vi "setUp.vi"(8 "error in (no error)":errorcluster, 11 "reference in":refnum<class "Engine Simulation Multi FPGA System Tests.lvclass">) -> (0 "error out":errorcluster, 3 "reference out":refnum<class "Engine Simulation Multi FPGA System Tests.lvclass">)   [LabVIEW 2017, in "Engine Simulation Multi FPGA System Tests.lvclass"]
doc: "setUp runs prior to the test method during test execution. Use this method to initialize any object data required by your tests."
uses:
  Engine Simulation Multi FPGA System Tests.lvclass
  C:/Program Files (x86)/National Instruments/LabVIEW 2017/vi.lib/addons/_JKI Toolkits/VI Tester/TestCase.llb/TestCase.lvclass
  <vilib>/addons/_JKI Toolkits/VI Tester/TestCase.llb/TestCase.lvclass
panel:
  in  "Minimum VeriStand Version":string="2017"
  in  "System Definition File":path=path "../Common Assets/EngineSimTest.nivssdf"
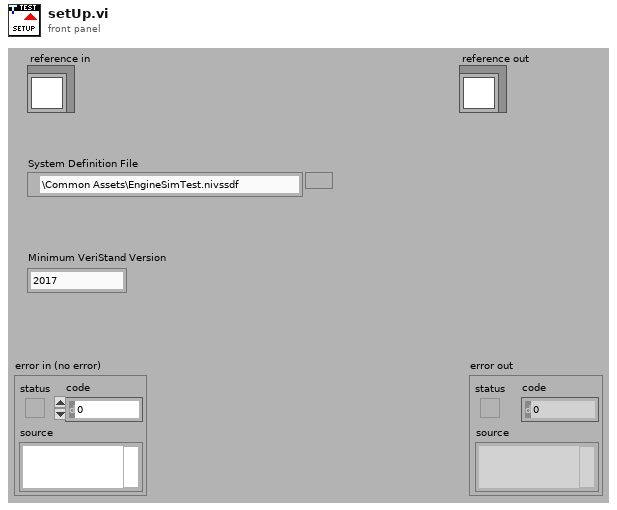
[diagram p1: front panel]
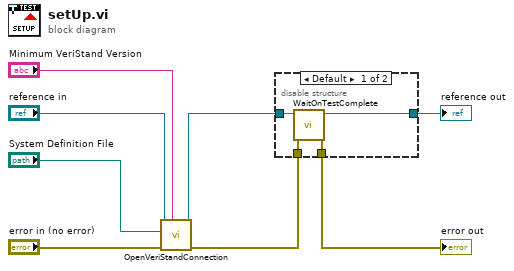
[diagram p0: block diagram]
diagram:
  n1 = call-dynamic "OpenVeriStandConnection.vi"("Minimum VeriStand Version (2016)"="Minimum VeriStand Version", "error in (no error)"="error in (no error)", "System Definition File"="System Definition File", "VeriStand Test Case in"="reference in") -> ("error out"=w2:errorcluster, "VeriStand Test Case out"=w3:refnum<class "Engine Simulation Multi FPGA System Tests.lvclass">)  [unwired: 5 in, 1 out]
  n2 = disable-structure shown="Default" {
    disable-tunnel: w2 -> [w12 w13]
    disable-tunnel: [w11 w13] -> w8
    disable-tunnel: [w10 w14] -> w7
    disable-tunnel: w3 -> [w9 w14]
    frame condition #0 (active) {
      n3 = call <vilib>:"WaitOnTestComplete.vi"("error in (no error)"=w12, "TestCase in"=w9) -> ("error out"=w11:errorcluster, "TestCase out"=w10:refnum<class "Engine Simulation Multi FPGA System Tests.lvclass">)  [unwired: 8 in]
    }
    frame condition #1 {
    }
  }
  "error out" <- w8
  "reference out" <- w7
